vi "Get Analysis ROI.vi"(11 "Analysis Graph in":refnum<class "Graph with Analysis Controls.lvclass">) -> (2 "ROI XYZ":T1, 3 "Analysis Graph out":refnum<class "Graph with Analysis Controls.lvclass">)   [LabVIEW 2023, in "Graph with Analysis Controls.lvclass"]
uses:
  Graph with Analysis Controls.lvclass
  D:/git/Lock-In-Thermography-Graphs/source/Series Graph/Graph with Series View.lvclass
  D:/git/Lock-In-Thermography-Graphs/source/Base Graph/Base Graph.lvclass
  Base Graph/Base Graph.lvclass/Base Graph.ctl
  Series Graph/Graph with Series View.lvclass/Graph with Series View.ctl
  Graph with Analysis Controls.lvclass/Graph with Analysis Controls.ctl
  Base Graph/Base Graph.lvclass
  Series Graph/Graph with Series View.lvclass
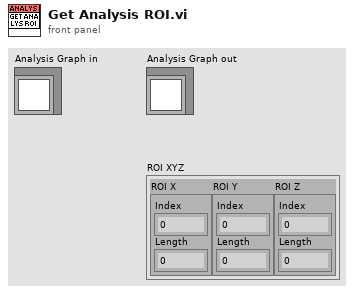
[diagram p1: front panel]
types:
  T1 = cluster{"ROI X":cluster{"Index":u32, "Length":u32}, "ROI Y":cluster{"Index":u32, "Length":u32}, "ROI Z":cluster{"Index":u32, "Length":u32}}
  T2 = cluster{"ROI X":cluster{"Index":u32, "Length":u32}, "ROI Y":cluster{"Index":u32, "Length":u32}}
  T3 = cluster{"ROI X":cluster{"Index":u32, "Length":u32}, "ROI Y":cluster{"Index":u32, "Length":u32}, "lower limit":cluster{"Index":u32, "Length":u32}}
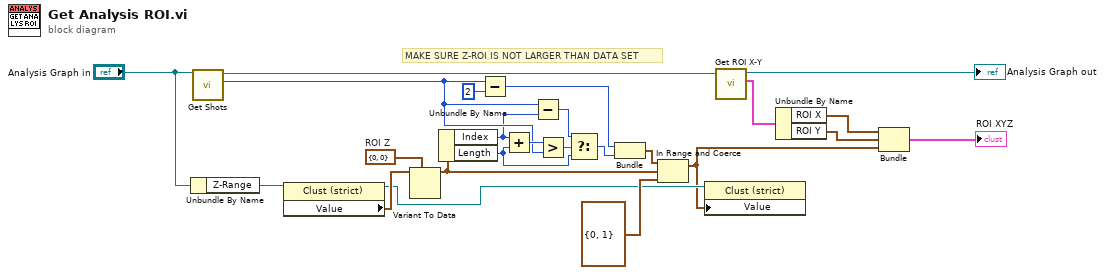
[diagram p0: block diagram]
diagram:
  w14 = cluster{"Index":u32, "Length":u32} {"Index"=0, "Length"=0}  # ROI Z
  # "MAKE SURE Z-ROI IS NOT LARGER THAN DATA SET"
  n1 = Unbundle By Name("Analysis Graph in") -> ("Z-Range"=w21:refnum<vi>)
  n2 = call "Get Shots.vi"("Series Graph in"="Analysis Graph in") -> ("Shots"=w7:u32, "Series Graph out"=w16:refnum<class "Graph with Analysis Controls.lvclass">)  [unwired: 9 in]
  n3 = property class="Clust (strict)"(reference=w21) -> (reference out=w3:refnum<vi>, "Value"=w17:cluster{"Index":u32, "Length":u32})  [unwired: 1 in, 1 out]
  n4 = Variant To Data(type=w14, Variant=w17) -> (data=w13:cluster{"Index":u32, "Length":u32})  [unwired: 1 in, 1 out]
  n5 = Unbundle By Name(w13) -> ("Index"=w1:u32, "Length"=w6:u32)
  n6 = Subtract(x=w7, y=u32 2) -> (x-y=w11:u32)
  n7 = Add(x=w1, y=w6) -> (x+y=w10:u32)
  n8 = Subtract(x=w7, y=w1) -> (x-y=w8:u32)
  n9 = Greater?(x=w10, y=w7) -> (0:w9:bool)
  n10 = Select(t=w8, s=w9, f=w6) -> (s? t:f=w5:u32)
  n11 = Bundle(w11, "Length"=w5) -> (w15:cluster{u32, "Length":u32})  [unwired: 1 in]
  n12 = In Range and Coerce(upper limit=w15, x=w13, lower limit=cluster{"Index":u32, "Length":u32} {"Index"=0, "Length"=1}) -> (coerced(x)=w2:cluster{"Index":u32, "Length":u32})  [unwired: 1 out]
  n13 = property class="Clust (strict)"(reference=w3, "Value"=w2) -> ()  [unwired: 1 in, 2 out]
  n14 = call "Get ROI X-Y.vi"("Base Graph in"=w16) -> ("ROI XY"=w20:T2, "Base Graph out"=→"Analysis Graph out":refnum<class "Graph with Analysis Controls.lvclass">)  [unwired: 9 in]
  n15 = Unbundle By Name(w20) -> ("ROI X"=w19:cluster{"Index":u32, "Length":u32}, "ROI Y"=w18:cluster{"Index":u32, "Length":u32})
  n16 = Bundle("ROI X"=w19, "ROI Y"=w18, "lower limit"=w2) -> (→"ROI XYZ":T3)  [unwired: 1 in]
